vi "Size of DataType.vi"(8 "error in":errorcluster, 11 "OD Entry in":refnum<class "OD Entry.lvclass">) -> (0 "error out":errorcluster, 2 "Size in Bits":i32, 3 "OD Entry out":refnum<class "OD Entry.lvclass">)   [LabVIEW 2024, in "Electronic Datasheet.lvlib" / "OD Entry.lvclass"]
doc: "Return the size in bits for the given CANopen datatype of this object, eg the size of what ever the datatype field is set to"
uses:
  OD Entry.lvclass
  OD Entry.lvclass/OD Entry.ctl
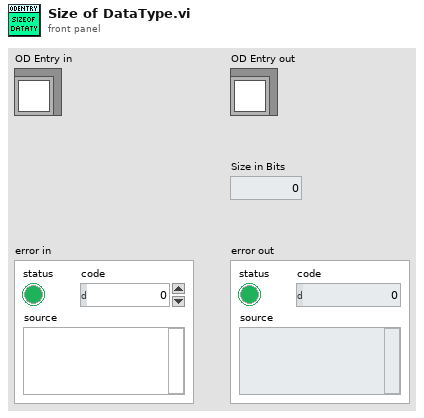
[diagram p1: front panel]
types:
  T1 = typedef "Electronic Datasheet.lvlib/Data Type.ctl" = u16
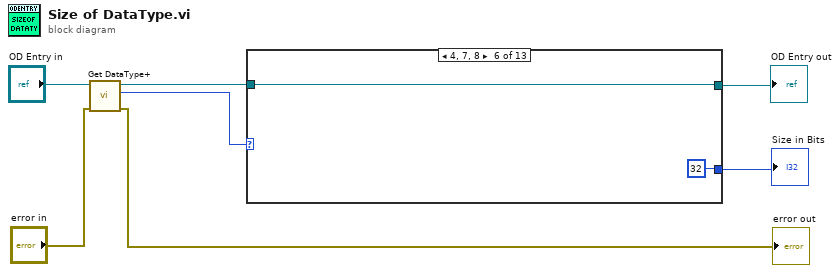
[diagram p0: block diagram]
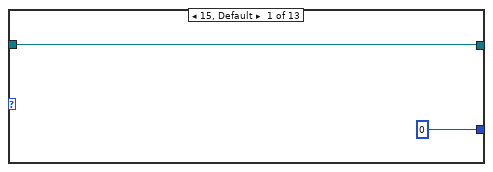
[diagram p2: hidden frame]
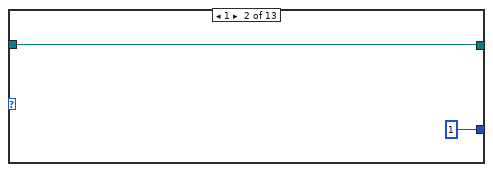
[diagram p3: hidden frame]
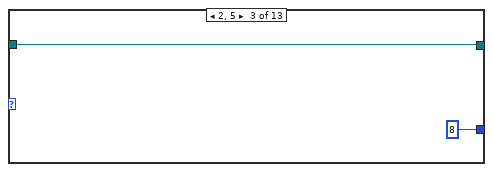
[diagram p4: hidden frame]
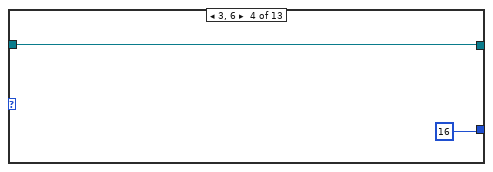
[diagram p5: hidden frame]
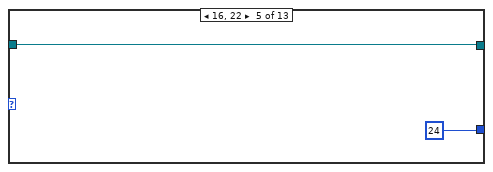
[diagram p6: hidden frame]
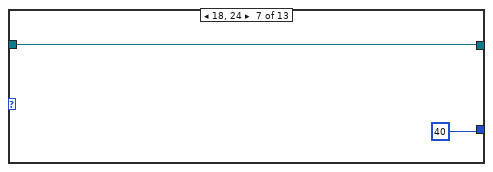
[diagram p7: hidden frame]
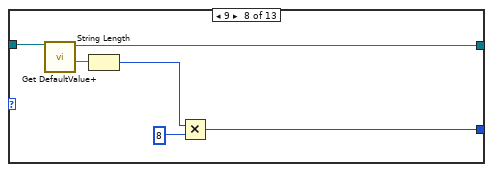
[diagram p8: hidden frame]
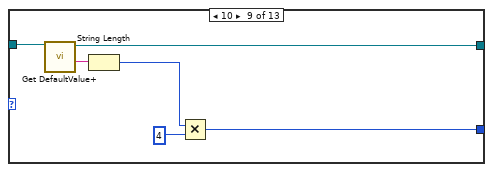
[diagram p9: hidden frame]
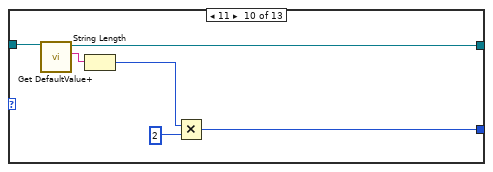
[diagram p10: hidden frame]
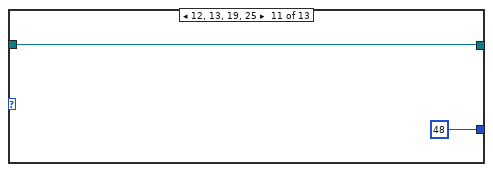
[diagram p11: hidden frame]
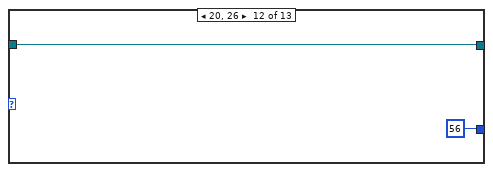
[diagram p12: hidden frame]
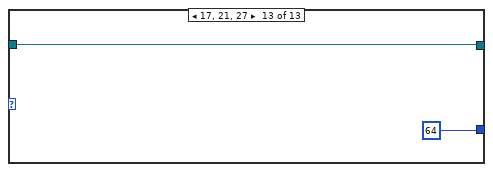
[diagram p13: hidden frame]
diagram:
  n1 = call "Get DataType+.vi"("Error In"="error in", "reference in"="OD Entry in") -> ("Error Out"=→"error out":errorcluster, "DataType"=w6:T1, "reference out"=w4:refnum<class "OD Entry.lvclass">)  [unwired: 6 in, 1 out]
  n2 = case shown="4, 7, 8" w6 {
    tunnel: [0 1 8 16 24 32 40 w27 w33 w34 48 56 64] -> w5
    tunnel: w4 -> [w8 w10 w12 w14 w16 w18 w20 w25 w31 w37 w40 w42 w44]
    tunnel: [w8 w10 w12 w14 w16 w18 w20 w22 w28 w36 w40 w42 w44] -> w3
    frame 15, Default {
      # "UNKNOWN"
    }
    frame 1 {
      # "BOOLEAN"
    }
    frame 2, 5 {
      # "INTEGER8"
    }
    frame 3, 6 {
      # "INTEGER16"
    }
    frame 16, 22 {
    }
    frame 4, 7, 8 {
      # "INTEGER32"
    }
    frame 18, 24 {
    }
    frame 9 {
      n3 = call "Get DefaultValue+.vi"("reference in"=w25) -> ("DefaultValue"=w24:string, "reference out"=w22:refnum<class "OD Entry.lvclass">)  [unwired: 7 in, 2 out]
      n4 = String Length(string=w24) -> (length=w23:i32)
      n5 = Multiply(x=w23, y=8) -> (x*y=w27:i32)
    }
    frame 10 {
      n6 = call "Get DefaultValue+.vi"("reference in"=w31) -> ("DefaultValue"=w30:string, "reference out"=w28:refnum<class "OD Entry.lvclass">)  [unwired: 7 in, 2 out]
      n7 = String Length(string=w30) -> (length=w29:i32)
      n8 = Multiply(x=w29, y=4) -> (x*y=w33:i32)
    }
    frame 11 {
      n9 = call "Get DefaultValue+.vi"("reference in"=w37) -> ("DefaultValue"=w35:string, "reference out"=w36:refnum<class "OD Entry.lvclass">)  [unwired: 7 in, 2 out]
      n10 = String Length(string=w35) -> (length=w38:i32)
      n11 = Multiply(x=w38, y=2) -> (x*y=w34:i32)
    }
    frame 12, 13, 19, 25 {
    }
    frame 20, 26 {
    }
    frame 17, 21, 27 {
    }
  }
  "OD Entry out" <- w3
  "Size in Bits" <- w5
